vi "facetrackeN.vi"() -> ()   [LabVIEW 2012]
uses:
  <userlib>/ImageProcessing/InitCamera_NTSC.vi
  <userlib>/ImageProcessing/LV86_Morph_Erosion.vi
  <userlib>/ImageProcessing/LV86_Morph_Dilation.vi
panel:
  out "Processed":picture
  in  "Cb2":cluster{i32, i32}(slide)={0, 3} scale=0.0..255.0
  in  "Cr 2":cluster{i32, i32}(slide)={0, 3} scale=0.0..255.0
  in  "Cb":cluster{i32, i32}(slide)={0, 3} scale=0.0..255.0
  out "Small Face":picture
  out "Compare Image":picture
  in  "Grab Image":bool
  out "image 4":picture
  in  "Cr":cluster{i32, i32}(slide)={0, 3} scale=0.0..255.0
  out "image 3":picture
  out "image 2":picture
  out "Cr":dbl[](array[numeric])
  out "Cb":dbl[](array[numeric])
  out "y":dbl[](array[numeric])
  out "image":picture
  in  "Stop":bool
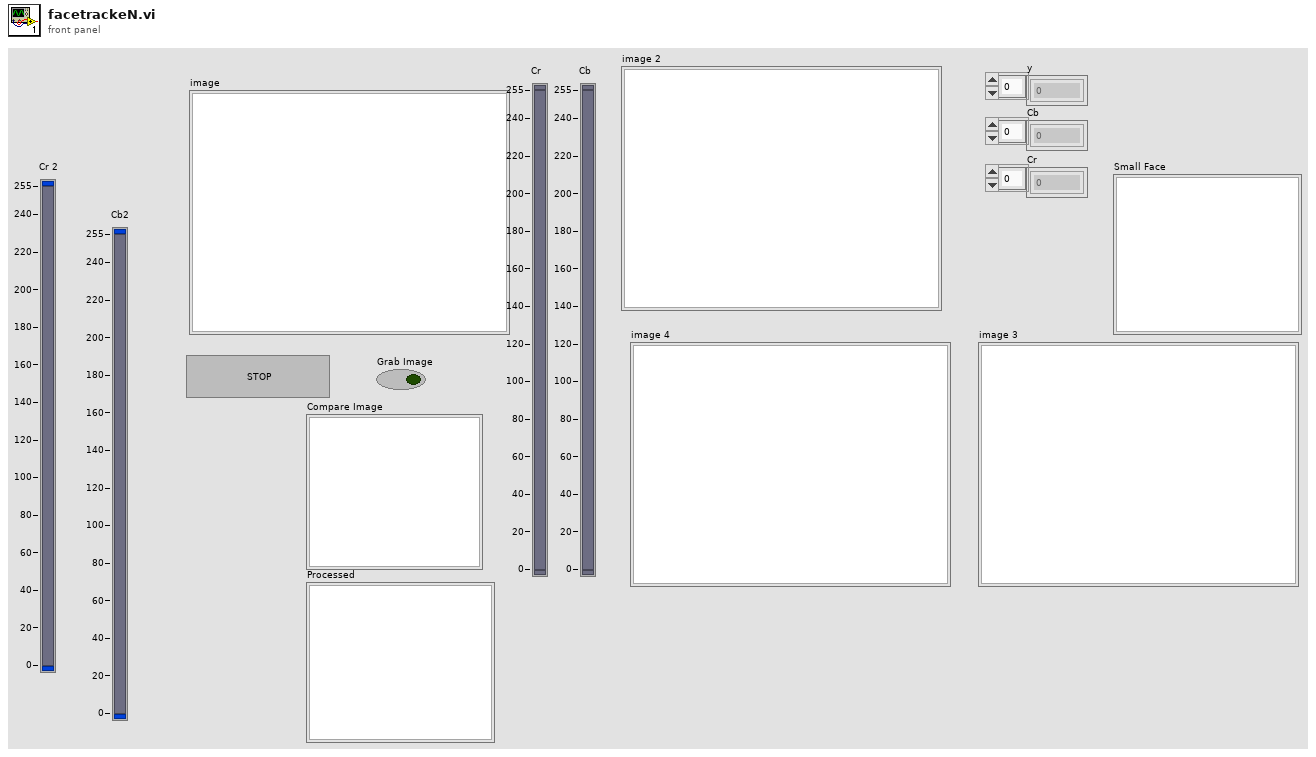
[diagram p1: front panel]
types:
  T1 = typedef "QT_Ref.ctl" = refnum<k1>
  T2 = cluster{"left":i16, "top":i16, "right":i16, "bottom":i16}
  T3 = typedef "QT_Image.ctl" = cluster{"Width":i32, "Height":i32, "Depth":i32, "data":u8[], "Compressed data":u8[], "Color table":u32[], "Duration":i32, "Options":i32, "Timestamp":i32, "ID":i32, "Reserved":i32, "Dialogs":u32}
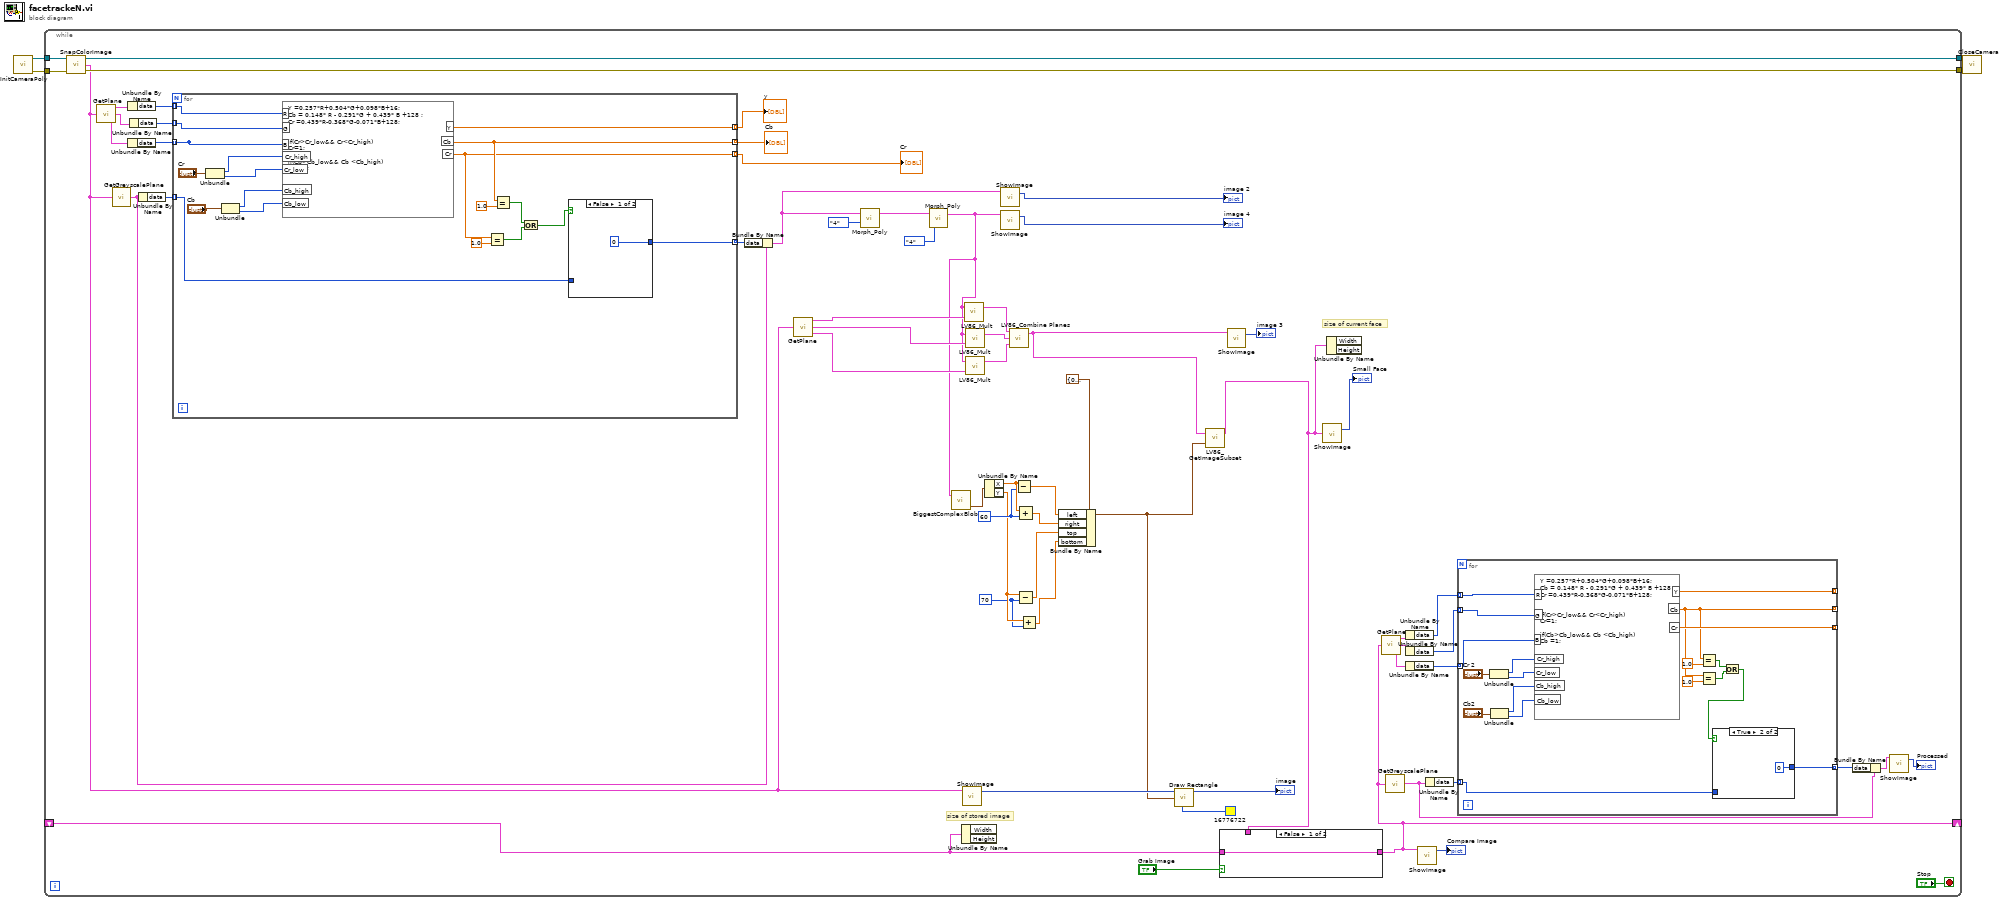
[diagram p0: block diagram]
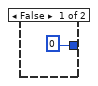
[diagram p2: hidden frame]
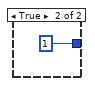
[diagram p4: hidden frame]
diagram:
  n1 = call-poly <userlib>:"InitCameraPoly.vi"() -> ("error out"=w1:errorcluster, "QT Ref Out"=w2:T1)  [unwired: 2 in]
  n2 = while {
    tunnel: w1 -> [w68]
    tunnel: w2 -> [w67]
    tunnel: [w66] -> w3
    tunnel: [w65] -> w4
    shift-right: [w11] -> _
    shift-left: _ -> [w36]
    stop <- "Stop" stop-if-true
    w23 = 60
    w20 = 70
    # "size of current face"
    # "size of stored image"
    n3 = call <userlib>:"SnapColorImage.vi"("error in (no error)"=w68, "QT Ref In"=w67) -> ("error out"=w66:errorcluster, "Image Out"=w35:T3, "QT Ref Out"=w65:T1)  [unwired: 1 in]
    n4 = call <userlib>:"GetPlane.vi"("Image In"=w35) -> ("Blue Plane Out"=w61:T3, "Green Plane Out"=w62:T3, "Red Plane Out"=w63:T3)
    n5 = call <userlib>:"GetGreyscalePlane.vi"("Image In"=w35) -> ("Greyscale  Out"=w50:T3)
    n6 = Unbundle By Name(w63) -> ("data"=w58:u8[])
    n7 = Unbundle By Name(w61) -> ("data"=w59:u8[])
    n8 = Unbundle By Name(w62) -> ("data"=w60:u8[])
    n9 = Unbundle By Name(w50) -> ("data"=w57:u8[])
    n10 = for {
      tunnel: w60 -> [w110] mode=indexing
      tunnel: [w109] -> _ mode=indexing
      tunnel: w59 -> [w109] mode=indexing
      tunnel: w58 -> [w108] mode=indexing
      tunnel: [w107] -> w55 mode=indexing
      tunnel: [w106] -> w54 mode=indexing
      tunnel: w57 -> [w99] mode=indexing
      tunnel: [w104] -> w53 mode=indexing
      tunnel: [w98] -> w52 mode=indexing
      n11 = Unbundle("Cr") -> (w97:i32, w96:i32)
      n12 = Unbundle("Cb") -> (w94:i32, w93:i32)
      n13 = formula code="Y =0.257*R+0.504*G+0.098*B+16;\nCb = 0.148* R - 0.291*G + 0.439* B +128 ;\nCr =0.439*R-0.368*G-0.071*B+128;\n\n\nif(Cr>Cr_low&& Cr<Cr_high)\nCr=1;\n\nif(Cb>Cb_low&& Cb <Cb_high)\nCb =1;"("G"=w110, "B"=w109, "R"=w108, "Cr_low"=w96, "Cr_high"=w97, "Cb_high"=w94, "Cb_low"=w93) -> ("Y"=w107:dbl, "Cb"=w106:dbl, "Cr"=w104:dbl)
      n14 = Equal?(x=w104, y=1.0) -> (x = y?=w101:bool)
      n15 = Equal?(x=w106, y=1.0) -> (x = y?=w102:bool)
      n16 = Or(x=w102, y=w101) -> (x .or. y?=w100:bool)
      n17 = case shown="False" w100 {
        tunnel: w99 -> [_ _]
        tunnel: [0 1] -> w98
        frame False {
        }
        frame True {
        }
      }
    }
    "y" <- w55
    "Cb" <- w54
    "Cr" <- w53
    n18 = Bundle By Name(cluster=w50, "data"=w52) -> (w32:T3)
    n19 = call <userlib>:"GetPlane.vi"("Image In"=w35) -> ("Blue Plane Out"=w47:T3, "Green Plane Out"=w48:T3, "Red Plane Out"=w49:T3)
    n20 = call-poly <userlib>:"Morph_Poly.vi"("Connectivity"=enum16{"4", "6", "8"}."4", "Image in"=w32) -> ("Image out"=w31:T3)  [unwired: 1 in]
    n21 = call-poly <userlib>:"Morph_Poly.vi"("Connectivity"=enum16{"4", "6", "8"}."4", "Image in"=w31) -> ("Image out"=w29:T3)  [unwired: 1 in]
    n22 = call <userlib>:"BiggestComplexBlob.vi"("Image in"=w29) -> ("Centroid"=w28:cluster{"X":dbl, "Y":dbl})  [unwired: 1 in, 2 out]
    n23 = Unbundle By Name(w36) -> ()  [unwired: 2 out]
    n24 = call <userlib>:"ShowImage.vi"("Image"=w35) -> ("image"=w42:picture)  [unwired: 2 in, 1 out]
    n25 = call <userlib>:"LV86_Mult.vi"("Image 2"=w49, "Image"=w29) -> ("Image Out"=w46:T3)  [unwired: 1 in]
    n26 = call <userlib>:"LV86_Mult.vi"("Image 2"=w48, "Image"=w29) -> ("Image Out"=w45:T3)  [unwired: 1 in]
    n27 = call <userlib>:"LV86_Mult.vi"("Image 2"=w47, "Image"=w29) -> ("Image Out"=w44:T3)  [unwired: 1 in]
    n28 = Unbundle By Name(w28) -> ("X"=w25:dbl, "Y"=w21:dbl)
    n29 = call <userlib>:"ShowImage.vi"("Image"=w32) -> ("image"=→"image 2":picture)  [unwired: 2 in, 1 out]
    n30 = call <userlib>:"ShowImage.vi"("Image"=w29) -> ("image"=→"image 4":picture)  [unwired: 2 in, 1 out]
    n31 = call <userlib>:"LV86_Combine Planes.vi"("Blue"=w44, "Green"=w45, "Red"=w46) -> ("Image 2"=w33:T3)  [unwired: 1 in]
    n32 = Subtract(x=w25, y=w23) -> (x-y=w26:dbl)
    n33 = Add(x=w25, y=w23) -> (x+y=w24:dbl)
    n34 = Subtract(x=w21, y=w20) -> (x-y=w22:dbl)
    n35 = Add(x=w21, y=w20) -> (x+y=w19:dbl)
    n36 = Bundle By Name(cluster=T2 {"left"=0, "top"=0, "right"=0, "bottom"=0} ("rect"), "left"=w26, "right"=w24, "top"=w22, "bottom"=w19) -> (w18:T2)
    n37 = call <vilib>:"Draw Rectangle.vi"("picture"=w42, "rect"=w18, "color(black)"=u32 16776722) -> ("new picture"=→"image":picture)  [unwired: 6 in]
    n38 = call <userlib>:"LV86_GetImageSubset.vi"("ROI"=w18, "Image In"=w33) -> ("Image out"=w9:T3)  [unwired: 1 in]
    n39 = case shown="False" "Grab Image" {
      tunnel: w36 -> [w90 _]
      tunnel: w9 -> [_ w91]
      tunnel: [w90 w91] -> w11
      frame False {
      }
      frame True {
        # "grab current image and save"
      }
    }
    n40 = call <userlib>:"ShowImage.vi"("Image"=w33) -> ("image"=→"image 3":picture)  [unwired: 2 in, 1 out]
    n41 = call <userlib>:"ShowImage.vi"("Image"=w9) -> ("image"=→"Small Face":picture)  [unwired: 2 in, 1 out]
    n42 = Unbundle By Name(w9) -> ()  [unwired: 2 out]
    n43 = call <userlib>:"GetPlane.vi"("Image In"=w11) -> ("Blue Plane Out"=w15:T3, "Green Plane Out"=w16:T3, "Red Plane Out"=w17:T3)
    n44 = call <userlib>:"GetGreyscalePlane.vi"("Image In"=w11) -> ("Greyscale  Out"=w7:T3)
    n45 = Unbundle By Name(w17) -> ("data"=w14:u8[])
    n46 = Unbundle By Name(w16) -> ("data"=w13:u8[])
    n47 = Unbundle By Name(w15) -> ("data"=w12:u8[])
    n48 = call <userlib>:"ShowImage.vi"("Image"=w11) -> ("image"=→"Compare Image":picture)  [unwired: 2 in, 1 out]
    n49 = Unbundle By Name(w7) -> ("data"=w10:u8[])
    n50 = for {
      tunnel: w14 -> [w87] mode=indexing
      tunnel: w13 -> [w86] mode=indexing
      tunnel: w12 -> [w85] mode=indexing
      tunnel: [w84] -> _ mode=indexing
      tunnel: [w82] -> _ mode=indexing
      tunnel: [w83] -> _ mode=indexing
      tunnel: w10 -> [w70] mode=indexing
      tunnel: [w69] -> w5 mode=indexing
      n51 = Unbundle("Cr 2") -> (w74:i32, w73:i32)
      n52 = Unbundle("Cb2") -> (w72:i32, w71:i32)
      n53 = formula code="Y =0.257*R+0.504*G+0.098*B+16;\nCb = 0.148* R - 0.291*G + 0.439* B +128 ;\nCr =0.439*R-0.368*G-0.071*B+128;\n\n\nif(Cr>Cr_low&& Cr<Cr_high)\nCr=1;\n\nif(Cb>Cb_low&& Cb <Cb_high)\nCb =1;"("R"=w87, "G"=w86, "B"=w85, "Cr_high"=w74, "Cr_low"=w73, "Cb_high"=w72, "Cb_low"=w71) -> ("Y"=w84:dbl, "Cb"=w82:dbl, "Cr"=w83:dbl)
      n54 = Equal?(x=w82, y=1.0) -> (x = y?=w81:bool)
      n55 = Equal?(x=w82, y=1.0) -> (x = y?=w80:bool)
      n56 = Or(x=w81, y=w80) -> (x .or. y?=w79:bool)
      n57 = case shown="True" w79 {
        tunnel: w70 -> [_ _]
        tunnel: [0 0] -> w69
        frame False {
        }
        frame True {
        }
      }
    }
    n58 = Bundle By Name(cluster=w7, "data"=w5) -> (w6:T3)
    n59 = call <userlib>:"ShowImage.vi"("Image"=w6) -> ("image"=→"Processed":picture)  [unwired: 2 in, 1 out]
  }
  n60 = call <userlib>:"CloseCamera.vi"("error in (no error)"=w3, "QT Ref In"=w4) -> ()  [unwired: 1 in, 1 out]
